vi "Build string table (word).vi"(6 "Graph data?":bool, 9 "row headers":string[](array[string]), 10 "column headers":string[](array[string]), 11 "text data":string[][](array[string])) -> (3 "output table":string[][](array[string]))   [LabVIEW 2010, in "NI_ReportGenerationToolkit.lvlib"]
uses:
  <vilib>/addons/_office/NI_ReportGenerationToolkit.lvlib
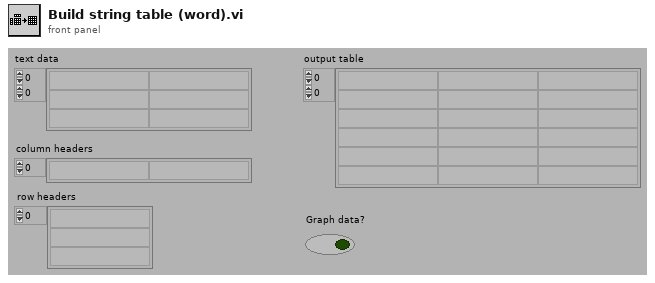
[diagram p1: front panel]
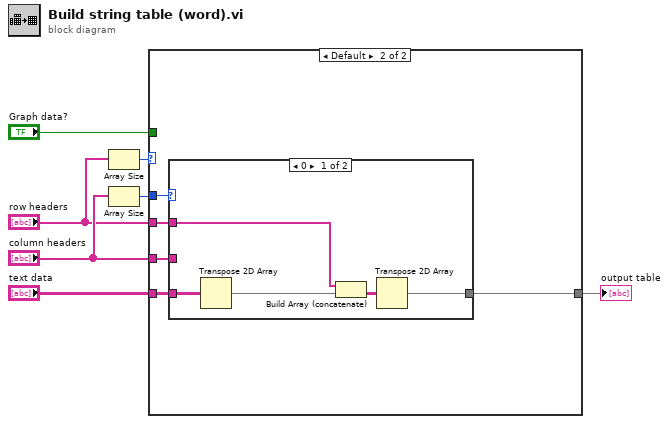
[diagram p0: block diagram]
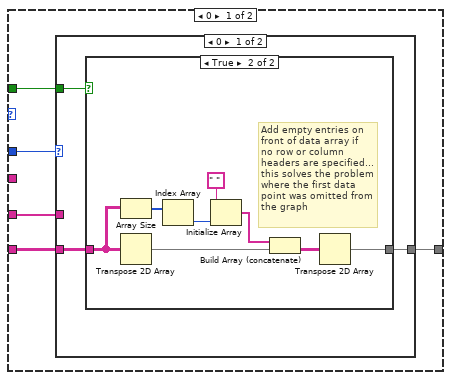
[diagram p2: hidden frame]
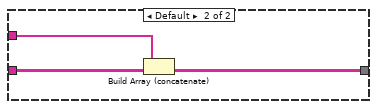
[diagram p4: hidden frame]
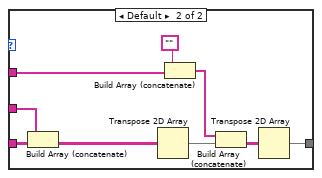
[diagram p5: hidden frame]
diagram:
  n1 = Array Size(array="row headers") -> (size(s)=w3:i32)
  n2 = Array Size(array="column headers") -> (size(s)=w2:i32)
  n3 = case shown="Default" w3 {
    tunnel: [w9 w32] -> w7
    tunnel: "column headers" -> [w11 w31]
    tunnel: w2 -> [w12 w30]
    tunnel: "text data" -> [w10 w29]
    tunnel: "row headers" -> [_ w28]
    tunnel: "Graph data?" -> [w8 _]
    frame 0 {
      n4 = case shown="0" w12 {
        tunnel: w11 -> [_ w27]
        tunnel: w10 -> [w14 w26]
        tunnel: [w15 w25] -> w9
        tunnel: w8 -> [w13 _]
        frame 0 {
          n5 = case shown="True" w13 {
            tunnel: [w16 w22] -> w15
            tunnel: w14 -> [w16 w18]
            frame False {
            }
            frame True {
              # "Add empty entries on\nfront of data array if\nno row or column \nheaders are specified...\nthis solves the problem\nwhere the first data \npoint was omitted from\nthe graph"
              n6 = Array Size(array=w18) -> (size(s)=w21:i32[])
              n7 = Transpose 2D Array(2D array=w18) -> (transposed array=w23:string[][])
              n8 = Index Array(array=w21) -> (element=w20:i32)  [unwired: 1 in]
              n9 = Initialize Array(" ", w20) -> (w17:string[])
              n10 = Build Array (concatenate)(w17, w23) -> (w24:string[][])
              n11 = Transpose 2D Array(2D array=w24) -> (transposed array=w22:string[][])
            }
          }
        }
        frame Default {
          n12 = Build Array (concatenate)(w27, w26) -> (w25:string[][])
        }
      }
    }
    frame Default {
      n13 = case shown="0" w30 {
        tunnel: [w34 w44] -> w32
        tunnel: w31 -> [_ w41]
        tunnel: w29 -> [w36 w40]
        tunnel: w28 -> [w37 w38]
        frame 0 {
          n14 = Transpose 2D Array(2D array=w36) -> (transposed array=w35:string[][])
          n15 = Build Array (concatenate)(w37, w35) -> (w33:string[][])
          n16 = Transpose 2D Array(2D array=w33) -> (transposed array=w34:string[][])
        }
        frame Default {
          n17 = Build Array (concatenate)(w41, w40) -> (w39:string[][])
          n18 = Transpose 2D Array(2D array=w39) -> (transposed array=w43:string[][])
          n19 = Build Array (concatenate)("", w38) -> (w42:string[])
          n20 = Build Array (concatenate)(w42, w43) -> (w45:string[][])
          n21 = Transpose 2D Array(2D array=w45) -> (transposed array=w44:string[][])
        }
      }
    }
  }
  "output table" <- w7
